vi "Get value form byte segment.vi"(3 "Input (HEX)":u8 format="0x%x", 4 "LSB":u8, 5 "MSB":u8) -> (1 "Value":u32)   [LabVIEW 2021]
panel:
  out "Value":bool[](array[boolean])
  out "Input":bool[](array[boolean])
  # "7"
  # "6"
  # "5"
  # "4"
  # "3"
  # "2"
  # "1"
  # "0"
  # "7"
  # "6"
  # "5"
  # "4"
  # "3"
  # "2"
  # "1"
  # "0"
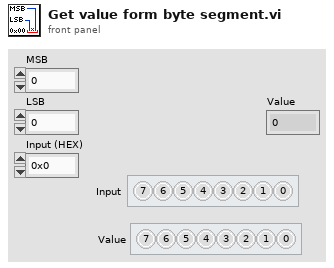
[diagram p1: front panel]
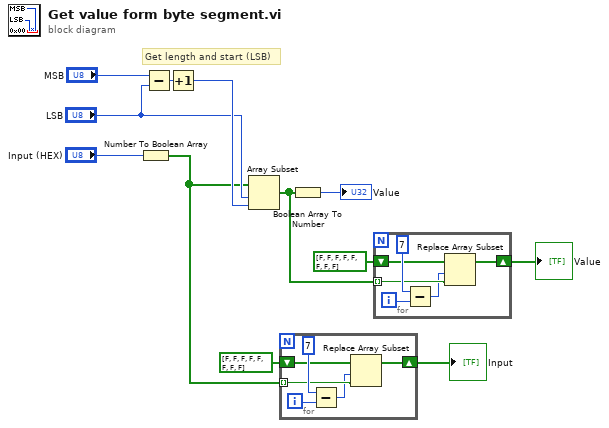
[diagram p0: block diagram]
diagram:
  # "Get length and start (LSB)"
  n1 = Number To Boolean Array(number="Input (HEX)") -> (Boolean array=w5:bool[])
  n2 = Subtract(x="MSB", y="LSB") -> (x-y=w12:u8)
  n3 = Increment(x=w12) -> (x+1=w11:u8)
  n4 = Array Subset(array=w5, index="LSB", length=w11) -> (w3:bool[])
  n5 = for {
    tunnel: w5 -> [w14] mode=indexing
    shift-right: [w15] -> w2
    shift-left: bool[] [FALSE, FALSE, FALSE, FALSE, FALSE, FALSE, FALSE, FALSE] ("array") -> [w16]
    i -> [w17]
    n6 = Subtract(x=7 ("y"), y=w17) -> (x-y=w13:i32)
    n7 = Replace Array Subset(array=w16, new element=w14, index=w13) -> (w15:bool[])
  }
  "Input" <- w2
  n8 = Boolean Array To Number(Boolean array=w3) -> (number=→"Value":u32)
  n9 = for {
    tunnel: w3 -> [w20] mode=indexing
    shift-right: [w21] -> w1
    shift-left: bool[] [FALSE, FALSE, FALSE, FALSE, FALSE, FALSE, FALSE, FALSE] ("array") -> [w22]
    i -> [w23]
    n10 = Subtract(x=7 ("y"), y=w23) -> (x-y=w19:i32)
    n11 = Replace Array Subset(array=w22, new element=w20, index=w19) -> (w21:bool[])
  }
  "Value" <- w1
